vi "Ex3-Select-Worksheet.vi"() -> ()   [LabVIEW 2021]
uses:
  <vilib>/Utility/NIReport.llb/Report Type.ctl
  <vilib>/Utility/NIReport.llb/NI_report.lvclass
  <vilib>/Utility/NIReport.llb/NI_ReportGenerationCore.lvlib
  <vilib>/Utility/NIReport.llb/Excel/NI_Excel.lvclass
  <vilib>/addons/_office/NI_ReportGenerationToolkit.lvlib
panel:
  out "Work sheet names":string[](array[string])
  out "Count":i32
  in  "file path (use dialog)":path
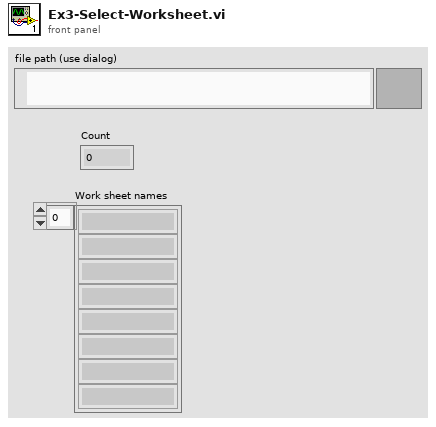
[diagram p1: front panel]
types:
  T1 = enum16{"open", "replace", "create", "open or create", "replace or create", "replace or create with confirmation"}
  T2 = typedef "NI_ReportGenerationCore.lvlib/Report Type.ctl" = enum16{"HTML", "Word", "Excel"}
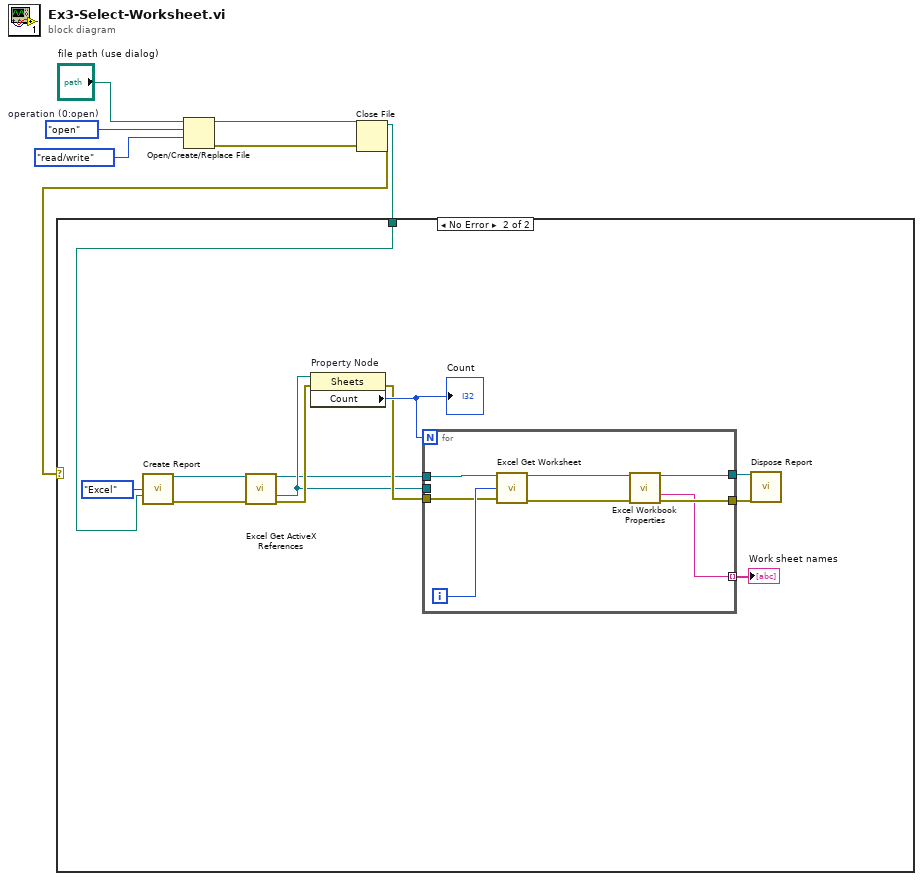
[diagram p0: block diagram]
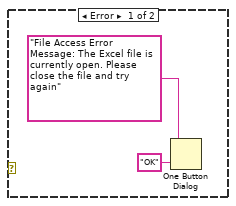
[diagram p2: hidden frame]
diagram:
  w4 = T1."open"  # operation (0:open)
  n1 = Open/Create/Replace File(file path (use dialog)="file path (use dialog)", operation (0:open)=w4, access (0:read/write)=enum16{"read/write", "read-only", "write-only"}."read/write") -> (refnum out=w7:refnum<file>, error out=w6:errorcluster)  [unwired: 3 in, 1 out]
  n2 = Close File(refnum=w7, error in=w6) -> (path=w1:path, error out=w2:errorcluster)
  n3 = case shown="No Error" w2 {
    tunnel: w1 -> [_ w20]
    frame Error {
      n4 = One Button Dialog(message="File Access Error Message: The Excel file is currently open. Please close the file and try again", button name ("OK")="OK") -> ()  [unwired: 1 out]
    }
    frame No Error {
      n5 = call <vilib>:"Create Report.vi"("report type"=Report_Type."Excel", "template (empty)"=w20) -> ("report out"=w19:refnum<class "NI_report.lvclass">, "error out"=w18:errorcluster)  [unwired: 12 in]
      n6 = call <vilib>:"Excel Get ActiveX References.vi"("report in"=w19, "error in (no error)"=w18) -> ("report out"=w13:refnum<class "NI_report.lvclass">, "Excel.Sheets"=w14:refnum<k7>, "error out"=w16:errorcluster)  [unwired: 7 in, 4 out]
      n7 = property on="Property Node" class="Sheets"(reference=w14, error in=w16) -> (error out=w15:errorcluster, "Count"=w17:i32)  [unwired: 1 out]
      "Count" <- w17
      n8 = for {
        N: w17 -> [_]
        tunnel: w15 -> [w23]
        tunnel: w14 -> [_]
        tunnel: w13 -> [w28]
        tunnel: [w26] -> w12
        tunnel: [w24] -> w11
        tunnel: [w22] -> w10 mode=indexing
        i -> [w29]
        n9 = call <vilib>:"Excel Get Worksheet.vi"("report in"=w28, "worksheet index (0)"=w29, "error in (no error)"=w23) -> ("report out"=w27:refnum<class "NI_report.lvclass">, "error out"=w25:errorcluster)  [unwired: 11 in]
        n10 = call <vilib>:"Excel Workbook Properties.vi"("report in"=w27, "error in (no error)"=w25) -> ("report out"=w26:refnum<class "NI_report.lvclass">, "current worksheet name"=w22:string, "error out"=w24:errorcluster)  [unwired: 10 in, 1 out]
      }
      "Work sheet names" <- w10
      n11 = call-dynamic "Dispose Report.vi"("report in"=w12, "error in (no error)"=w11) -> ()  [unwired: 13 in, 1 out]
    }
  }
